vi "merFISH_autofocus_signal_search.vi"(5 "queue ASI stage":refnum<queue>, 6 "error in":errorcluster, 7 "Search range":i32=-25, 8 "Slope":dbl, 9 "QPD ref":T1) -> (0 "error out":errorcluster, 3 "Ref found?":bool)   [LabVIEW 2015]
uses:
  CONTROLS/Q_ASI_stage_element.ctl
  <vilib>/Utility/miscctls.llb/LVCursorListTypeDef.ctl
  GLOBAL/Global_ASI_stage.vi
  GLOBAL/Global_FPGA.vi
panel:
  out "XY Graph":cluster{"X":dbl, "Y":dbl}[](graph)
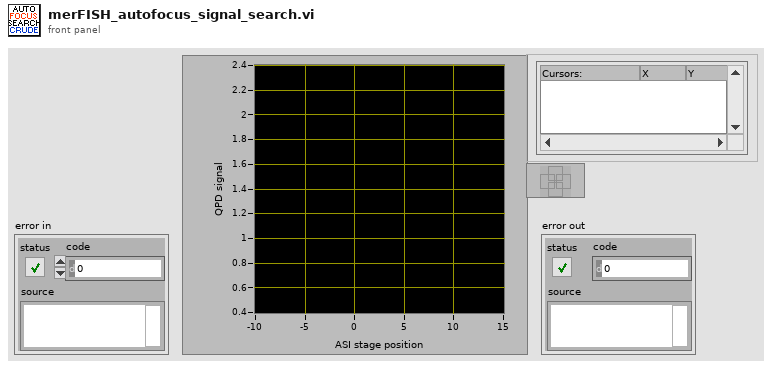
[diagram p1: front panel]
types:
  T1 = cluster{"X":sgl, "Y":sgl, "SUM":sgl, "count":u32}
  T2 = typedef "Q_ASI_stage_element.ctl" = cluster{"variant":variant, "Instruction":enum16{"ASI_idle", "ASI_initialize", "ASI_error", "ASI_security_stop", "ASI_read_XYZ", "ASI_up", "ASI_down", "ASI_left", "ASI_right", "ASI_save_XY", "ASI_move_to_XY", "ASI_brightfield", "ASI_init_scan", "ASI_init_merFISH", "ASI_move_to_XY_merFISH", "ASI_move_to_Z_merFISH", "ASI_init_autofocus_search_merFISH", "ASI_close_autofocus_search_merFISH", "ASI_adjust_piezo_autofocus_merFISH", "ASI_set_piezo_autofocus_to_reference_position_merFISH_TL", "ASI_close_merFISH", "ASI_stop"}}
  T3 = typedef "LVCursorListTypeDef.ctl" = cluster{"Name":string, "Color":u32, "Style":u8, "Point Style":u8, "Name Visible":bool, "Allow Drag":bool, "Cursor Mode":u32, "Plot":i32, "Index":i32, "Position":cluster{"X":dbl, "Y":dbl}, "X Scale":u32, "Y Scale":u32, "Watch Plots":i32[], "Watch All Plots":bool, "Plot Area":i32, "Label Offset":cluster{"X":dbl, "Y":dbl}}[]
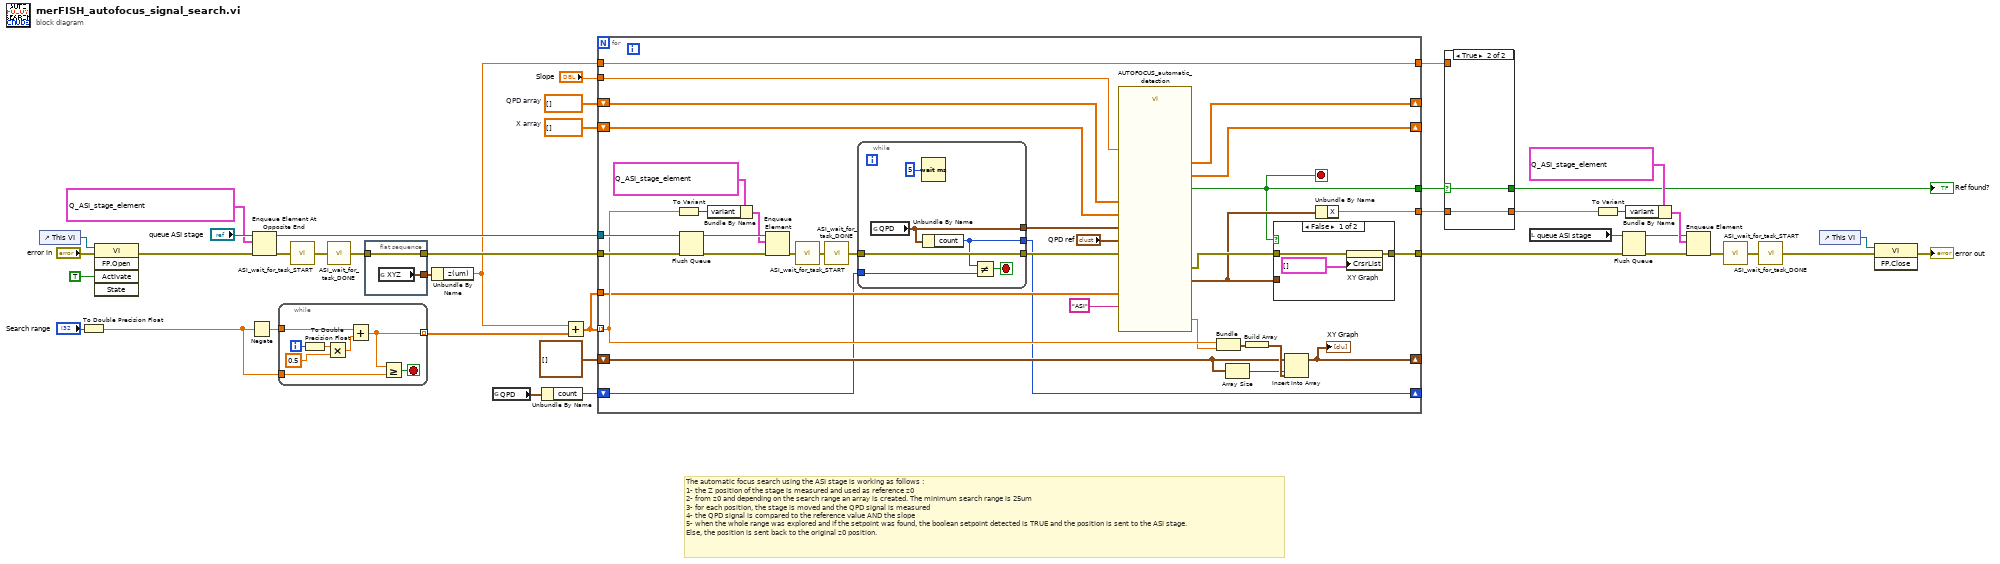
[diagram p0: block diagram]
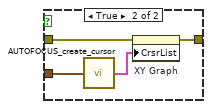
[diagram p3: hidden frame]
diagram:
  w12 = dbl[] []  # QPD array
  w13 = dbl[] []  # X array
  # "The automatic focus search using the ASI stage is working as follows :\n1- the Z position of the stage is measured and used as reference z0\n2- from z0 and depending on the search range an array is created. The minimum search range is 25um\n3- for each position, the stage is moved and the QPD signal is measured\n4- the QPD signal is compared to the reference value AND the slope\n5- when the whole range was explored and if the setpoint was found, the boolean setpoint detected is TRUE and the position is sent to the ASI stage.\nElse, the position is sent back to the original z0 position."
  n1 = control-ref of="This VI"() -> (w22:refnum<vi>)
  n2 = To Double Precision Float(number="Search range") -> (double precision float=w14:dbl)
  n3 = invoke class="VI" method="FP.Open"(reference=w22, error in="error in", "Activate"=TRUE ("Activate?")) -> (error out=w20:errorcluster)  [unwired: 2 in, 4 out]
  n4 = Negate(x=w14) -> (-x=w15:dbl)
  n5 = Enqueue Element At Opposite End(queue="queue ASI stage", element=T2 {"variant"=variant, "Instruction"=enum."ASI_init_autofocus_search_merFISH"}, error in (no error)=w20) -> (queue out=w34:refnum<queue>, error out=w39:errorcluster)  [unwired: 1 in, 1 out]
  n6 = while {
    tunnel: w15 -> [w46]
    tunnel: [w44] -> w35 mode=indexing
    tunnel: w14 -> [w42]
    i -> [w49]
    stop <- w43 stop-if-true
    n7 = To Double Precision Float(number=w49) -> (double precision float=w47:dbl)
    n8 = Multiply(x=w47, y=0.5) -> (x*y=w45:dbl)
    n9 = Add(x=w46, y=w45) -> (x+y=w44:dbl)
    n10 = Greater Or Equal?(x=w44, y=w42) -> (x >= y?=w43:bool)
  }
  n11 = call "ASI_wait_for_task_START.vi"("error in"=w39) -> ("error out"=w38:errorcluster)
  n12 = call "ASI_wait_for_task_DONE.vi"("error in"=w38) -> ("error out"=w37:errorcluster)
  n13 = flat-sequence {
    tunnel: w37 -> [w51]
    tunnel: [w51] -> w33
    tunnel: [w50] -> w36
    frame #0 {
      n14 = global read "Global_ASI_stage.vi" "XYZ"() -> (w50:cluster{"x(um)":dbl, "y(um)":dbl, "z(um)":dbl})
    }
  }
  n15 = Unbundle By Name(w36) -> ("z(um)"=w8:dbl)
  n16 = global read "Global_FPGA.vi" "QPD"() -> (w2:T1)
  n17 = Unbundle By Name(w2) -> ("count"=w1:u32)
  n18 = Add(x=w8, y=w35) -> (x+y=w11:dbl[])
  n19 = for {
    tunnel: w11 -> [w72] mode=indexing
    tunnel: w34 -> [w86]
    tunnel: w33 -> [w73]
    shift-right: [w75] -> _
    shift-left: cluster{dbl, "norm":dbl}[] [] ("appended array") -> [w76]
    tunnel: [w65] -> w10
    shift-right: [w69] -> _
    shift-left: w13 -> [w70]
    shift-right: [w67] -> _
    shift-left: w12 -> [w68]
    tunnel: w11 -> [w64]
    tunnel: [w59] -> w7
    tunnel: [w62] -> w6
    tunnel: "Slope" -> [w61]
    tunnel: w8 -> [w60]
    tunnel: [w60] -> w4
    shift-right: [w52] -> _
    shift-left: w1 -> [w53]
    stop <- w59 stop-if-true
    n20 = To Variant(anything=w72) -> (Variant=w81:variant)
    n21 = Flush Queue(queue=w86, error in (no error)=w73) -> (queue out=w85:refnum<queue>, error out=w84:errorcluster)  [unwired: 1 out]
    n22 = Bundle By Name(cluster=T2 {"variant"=variant, "Instruction"=enum."ASI_move_to_Z_merFISH"} ("element"), "variant"=w81) -> (w82:T2)
    n23 = Enqueue Element(queue=w85, element=w82, error in (no error)=w84) -> (error out=w80:errorcluster)  [unwired: 1 in, 2 out]
    n24 = call "ASI_wait_for_task_START.vi"("error in"=w80) -> ("error out"=w79:errorcluster)
    n25 = call "ASI_wait_for_task_DONE.vi"("error in"=w79) -> ("error out"=w57:errorcluster)
    n26 = while {
      tunnel: w57 -> [w92]
      tunnel: [w92] -> w55
      tunnel: w53 -> [w90]
      tunnel: [w89] -> w56
      tunnel: [w87] -> w52
      stop <- w88 stop-if-true
      n27 = global read "Global_FPGA.vi" "QPD"() -> (w89:T1)
      n28 = Wait (ms)(milliseconds to wait=u32 5) -> ()  [unwired: 1 out]
      n29 = Unbundle By Name(w89) -> ("count"=w87:u32)
      n30 = Not Equal?(x=w87, y=w90) -> (x != y?=w88:bool)
    }
    n31 = call "AUTOFOCUS_automatic_detection.vi"("X array"=w70, "QPD array"=w68, "Stage type"="ASI", "QPD ref"="QPD ref", "Slope"=w61, "QPD"=w56, "error in"=w55, "Search array"=w64) -> ("QPD array out"=w67:dbl[], "X array out"=w69:dbl[], "Cursor"=w63:cluster{"X":dbl, "Y":dbl}, "Setpoint detected"=w59:bool, "norm"=w71:dbl, "error out"=w66:errorcluster)  [unwired: 2 in]
    n32 = Bundle(w72, "norm"=w71) -> (w78:cluster{dbl, "norm":dbl})  [unwired: 1 in]
    n33 = Array Size(array=w76) -> (size(s)=w74:i32)
    n34 = Build Array(w78) -> (w77:cluster{dbl, "norm":dbl}[])
    n35 = case shown="False" w59 {
      tunnel: w66 -> [w95 w98]
      tunnel: [w94 w97] -> w65
      tunnel: w63 -> [_ w99]
      frame False {
        n36 = property on="XY Graph" class="XYGraph (strict)"(error in=w95, "CrsrList"=T3 [] ("Cursor List")) -> (error out=w94:errorcluster)  [unwired: 1 in, 1 out]
      }
      frame True {
        n37 = call "AUTOFOCUS_create_cursor.vi"("Position"=w99) -> ("cursor array"=w96:T3)
        n38 = property on="XY Graph" class="XYGraph (strict)"(error in=w98, "CrsrList"=w96) -> (error out=w97:errorcluster)  [unwired: 1 in, 1 out]
      }
    }
    n39 = Insert Into Array(array=w76, index=w74, new element=w77) -> (w75:cluster{dbl, "norm":dbl}[])
    "XY Graph" <- w75
    n40 = Unbundle By Name(w63) -> ("X"=w62:dbl)
  }
  n41 = case shown="True" w7 {
    selector: w7 -> [w101 w102]
    tunnel: w6 -> [_ w103]
    tunnel: [w100 w103] -> w5
    tunnel: w4 -> [w100 _]
    tunnel: [w101 w102] -> w3
    frame False {
    }
    frame True {
    }
  }
  "Ref found?" <- w3
  n42 = local read "queue ASI stage"() -> (w24:refnum<queue>)
  n43 = To Variant(anything=w5) -> (Variant=w29:variant)
  n44 = Flush Queue(queue=w24, error in (no error)=w10) -> (queue out=w25:refnum<queue>, error out=w26:errorcluster)  [unwired: 1 out]
  n45 = Bundle By Name(cluster=T2 {"variant"=variant, "Instruction"=enum."ASI_move_to_Z_merFISH"} ("element"), "variant"=w29) -> (w28:T2)
  n46 = Enqueue Element(queue=w25, element=w28, error in (no error)=w26) -> (error out=w30:errorcluster)  [unwired: 1 in, 2 out]
  n47 = call "ASI_wait_for_task_START.vi"("error in"=w30) -> ("error out"=w31:errorcluster)
  n48 = call "ASI_wait_for_task_DONE.vi"("error in"=w31) -> ("error out"=w18:errorcluster)
  n49 = control-ref of="This VI"() -> (w19:refnum<vi>)
  n50 = invoke class="VI" method="FP.Close"(reference=w19, error in=w18) -> (error out=→"error out":errorcluster)  [unwired: 1 in, 2 out]
